vi "Set Algorithm Parameters.vi"(7 "Dimension":i32, 8 "error in (no error)":errorcluster, 9 "Number of Generations":i32, 10 "Front Panel Menu":T1={"Crossover Probability"=0.75, "Mutation Probability"=0.2, "Population Size"=80, "Strategy"=enum."Total Replacement", "Plot Type"=enum."No Plot", "Crossover Type"=enum."One Point Cx", "Mutation Type"=enum."Swap", "Scheduler"=enum."Non Delay Scheduler", "Reorder"=FALSE, "Objective "=enum."Makespan", "Local Search "=enum."No Local Search", "Initial Population Generation"=enum."Random"}, 11 "GA in":refnum<class "GA.lvclass">) -> (0 "error out":errorcluster, 3 "GA out":refnum<class "GA.lvclass">)   [LabVIEW 2013, in "GA.lvclass"]
uses:
  GA.lvclass
  Controls/Front Panle Menu.ctl
  Controls/Strategy.ctl
  Controls/Plot Type.ctl
  Controls/Crossover Type.ctl
  Controls/Mutation Type.ctl
  GA/Controls/Scheduler Type.ctl
  GA/Controls/Objective.ctl
  GA/Controls/Local Search Type.ctl
  Controls/Initial Population Generation.ctl
  Controls/Solution_GA.ctl
  Controls/Population Statistics.ctl
  GA.lvclass/GA.ctl
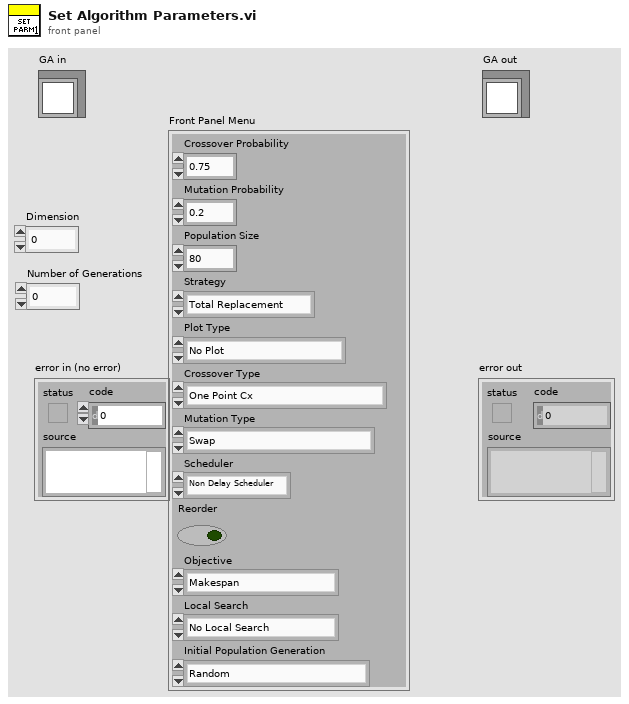
[diagram p1: front panel]
types:
  T1 = typedef "Front Panle Menu.ctl" = cluster{"Crossover Probability":dbl, "Mutation Probability":dbl, "Population Size":u8, "Strategy":T2, "Plot Type":T3, "Crossover Type":T4, "Mutation Type":T5, "Scheduler":T6, "Reorder":bool, "Objective ":T7, "Local Search ":T8, "Initial Population Generation":T9}
  T2 = typedef "Strategy.ctl" = enum16{"Total Replacement", "Incremental Replacement", "Ellitist 1", "Elitist 2", "%10", "%20", "%30", "%40", "%50"}
  T3 = typedef "Plot Type.ctl" = enum16{"No Plot", "Min Max Mean Plot", "Gannt Chart"}
  T4 = typedef "GA.lvclass/Crossover Type.ctl" = enum16{"One Point Cx", "Two Point Cx", "Ordered Cx (OX)", "Linear Order Cx (LOX)", "Cycle Cx", "Specialized Cx", "JO4M Cx", "MPOX1", "MPOX1 Random", "MPOX2", "MPOX2 Random"}
  T5 = typedef "GA.lvclass/Mutation Type.ctl" = enum16{"Swap", "Non-Redundant Swap", "Insert", "Shift", "Shuflle", "Inversion", "SA", "IRH3T", "JO4M Swap", "MO4J Swap", "SPT JO4M", "LCTJ Swap", "Low's Mutation", "ND Mutation"}
  T6 = typedef "Scheduler Type.ctl" = enum16{"Non Delay Scheduler", "GT Active Scheduler", "FIFO Scheduler"}
  T7 = typedef "Objective.ctl" = enum16{"Makespan", "Total Tardiness"}
  T8 = typedef "Local Search Type.ctl" = enum16{"No Local Search", "SA Population", "IRH3T(Pop)", "IRH3T(Best Solution)", "SA Best Solution", "SA Random Solution", "SA Random 3 Solutions", "SA Hybrid", "VNS Best Solution", "VNS Random Solution"}
  T9 = typedef "GA.lvclass/Initial Population Generation.ctl" = enum16{"Random", "Heuristic Solution"}
  T10 = typedef "Population Statistics.ctl" = cluster{"Min":u16, "Max":u16, "Mean":dbl}
  T11 = typedef "Solution_GA.ctl" = cluster{"Schedule":u16[], "Fitness":u16, "Fitness Valid?":bool}
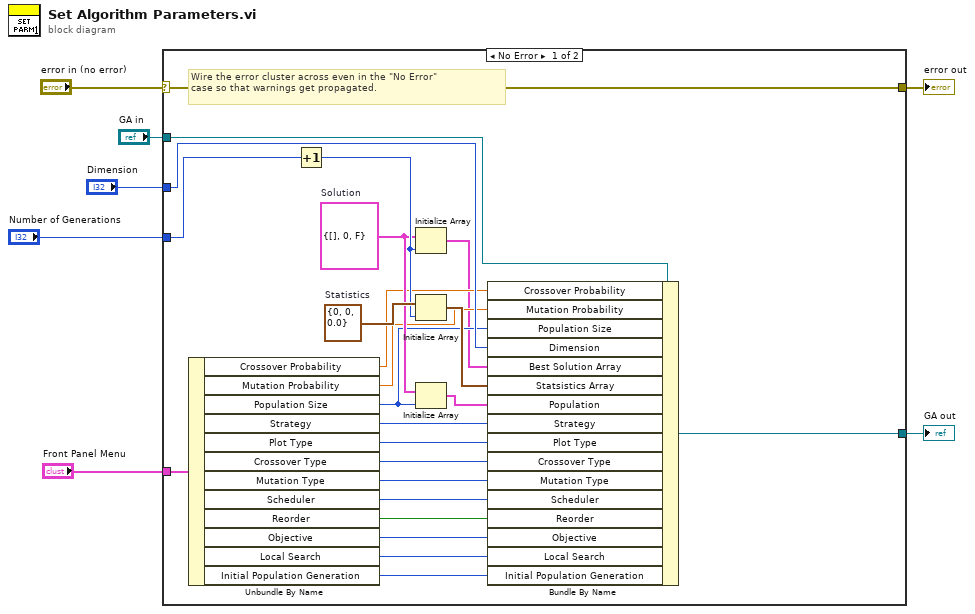
[diagram p0: block diagram]
diagram:
  n1 = case shown="No Error" "error in (no error)" {
    selector: "error in (no error)" -> [w31 w33]
    tunnel: [w31 w33] -> w6
    tunnel: [w29 w32] -> w4
    tunnel: "GA in" -> [w30 w32]
    tunnel: "Dimension" -> [w28 _]
    tunnel: "Number of Generations" -> [w25 _]
    tunnel: "Front Panel Menu" -> [w21 _]
    frame No Error {
      w27 = T10 {"Min"=0, "Max"=0, "Mean"=0.0}  # Statistics
      w23 = T11 {"Schedule"=[], "Fitness"=0, "Fitness Valid?"=FALSE}  # Solution
      # "Wire the error cluster across even in the \"No Error\"\ncase so that warnings get propagated."
      n2 = Unbundle By Name(w21) -> ("Crossover Probability"=w20:dbl, "Mutation Probability"=w19:dbl, "Population Size"=w18:u8, "Strategy"=w17:T2, "Plot Type"=w16:T3, "Crossover Type"=w15:T4, "Mutation Type"=w14:T5, "Scheduler"=w13:T6, "Reorder"=w12:bool, "Objective"=w11:T7, "Local Search"=w9:T8, "Initial Population Generation"=w8:T9)
      n3 = Increment(x=w25) -> (x+1=w24:i32)
      n4 = Initialize Array(w23, w24) -> (w10:T11[])
      n5 = Initialize Array(w27, w24) -> (w26:T10[])
      n6 = Initialize Array(w23, w18) -> (w22:T11[])
      n7 = Bundle By Name(cluster=w30, "Crossover Probability"=w20, "Mutation Probability"=w19, "Population Size"=w18, "Dimension"=w28, "Best Solution Array"=w10, "Statsistics Array"=w26, "Population"=w22, "Strategy"=w17, "Plot Type"=w16, "Crossover Type"=w15, "Mutation Type"=w14, "Scheduler"=w13, "Reorder"=w12, "Objective"=w11, "Local Search"=w9, "Initial Population Generation"=w8) -> (w29:refnum<class "GA.lvclass">)
    }
    frame Error {
    }
  }
  "error out" <- w6
  "GA out" <- w4
